vi "OnDataChange.vi"(0 "DemoStepMotor in":refnum<class "DemoStepMotor.lvclass">, 1 "DataExchange":T1, 3 "error in (no error)":errorcluster) -> (7 "DemoStepMotor out":refnum<class "DemoStepMotor.lvclass">, 10 "error out":errorcluster)   [LabVIEW 2020, in "DemoStepMotor.lvlib" / "DemoStepMotor.lvclass"]
uses:
  DemoStepMotor.lvclass
  Hardware Abstraction Layer/Component/Device/Device/DataExchange.ctl
  <vilib>/vision/Image Controls.llb/IMAQ Image.ctl
  DemoStepMotor.lvclass/DemoStepMotor.ctl
  Interface/DataListener Messages/OnDataChange Msg/OnDataChange Msg.lvclass/OnDataChange Msg.ctl
  <vilib>/ActorFramework/Message Enqueuer/Message Enqueuer.lvclass/Message Enqueuer.ctl
  <vilib>/ActorFramework/Message Enqueuer/Enqueue.vi
  Interface/DataListener Messages/OnDataChange Msg/OnDataChange Msg.lvclass
  C:/Program Files/National Instruments/LabVIEW 2020/vi.lib/ActorFramework/Message/Message.lvclass
  <vilib>/ActorFramework/Message Priority Queue/Priority Enqueue.vi
  Hardware Abstraction Layer/Component/Stage/Stage/Stage.lvclass
  Interface/DataListener/DataListener.lvclass
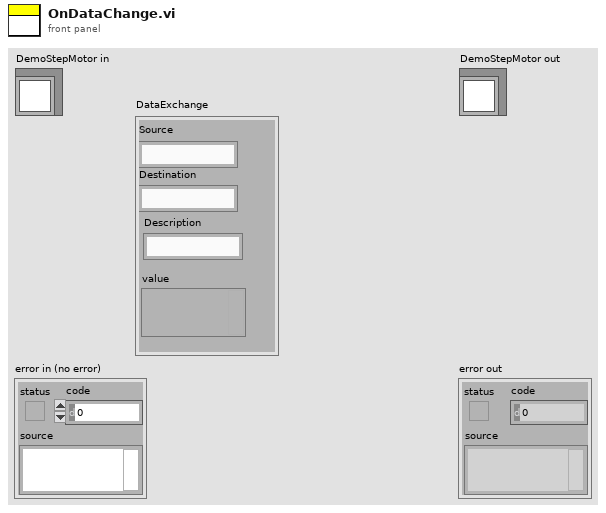
[diagram p1: front panel]
types:
  T1 = typedef "DataListener.lvclass/DataExchange.ctl" = cluster{"Source":string, "Destination":string, "Description":string, "value":variant}
  T2 = typedef "IMAQ Image.ctl" = refnum<image>
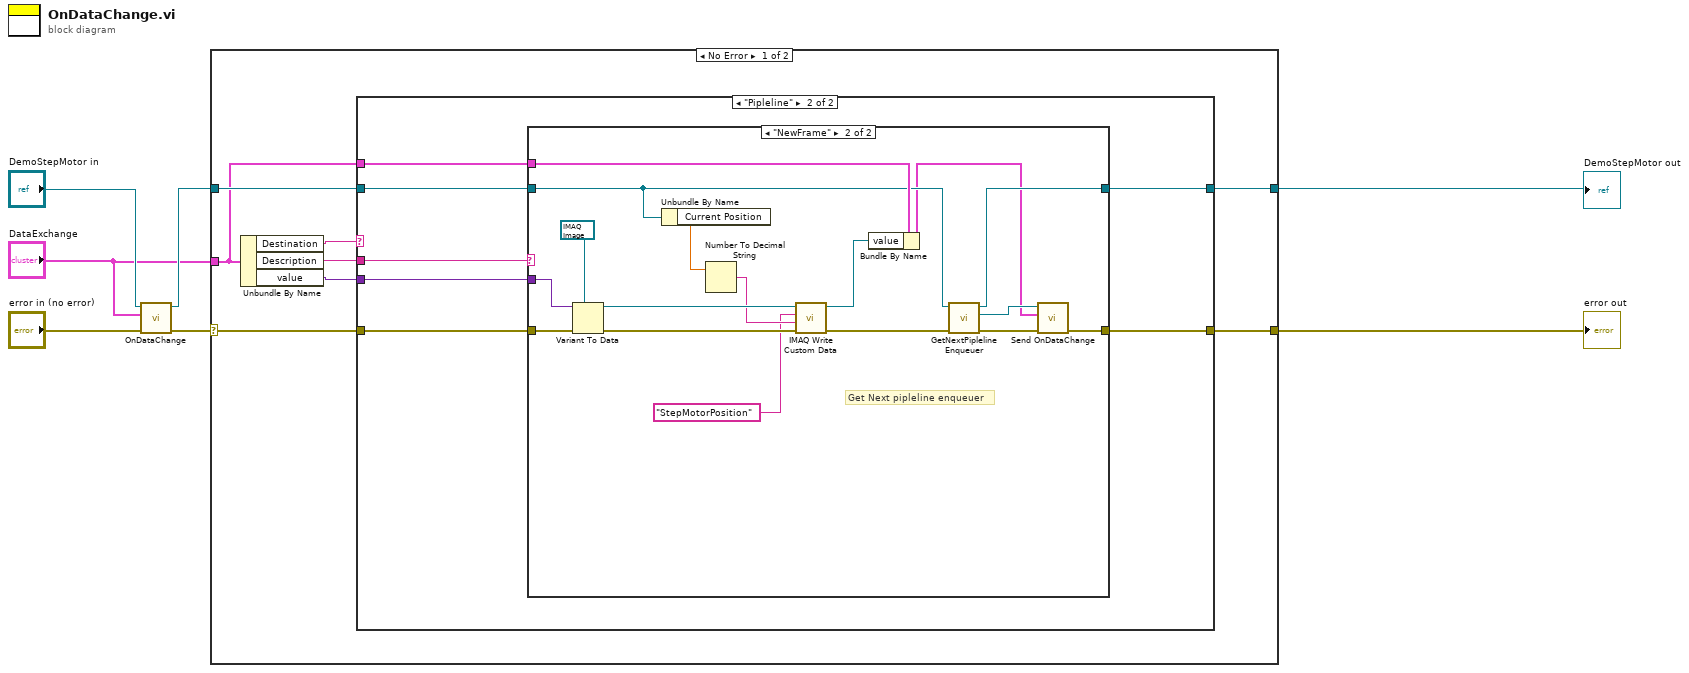
[diagram p0: block diagram]
diagram:
  n1 = call-parent "OnDataChange.vi"("Device in"="DemoStepMotor in", "DataExchange"="DataExchange", "error in (no error)"="error in (no error)") -> ("Device out"=w3:refnum<class "DemoStepMotor.lvclass">, "error out"=w5:errorcluster)  [unwired: 6 in]
  n2 = case shown="No Error" w5 {
    selector: w5 -> [w11 w45]
    tunnel: [w12 w45] -> w4
    tunnel: w3 -> [w14 w44]
    tunnel: [w13 w44] -> w2
    tunnel: "DataExchange" -> [w8 _]
    frame No Error {
      n3 = Unbundle By Name(w8) -> ("Destination"=w15:string, "Description"=w10:string, "value"=w9:variant)
      n4 = case shown="\"Pipleline\"" w15 {
        tunnel: [w17 w22] -> w13
        tunnel: w14 -> [w17 w21]
        tunnel: [w16 w19] -> w12
        tunnel: w11 -> [w16 w20]
        tunnel: w10 -> [_ w24]
        tunnel: w9 -> [_ w23]
        tunnel: w8 -> [_ w18]
        frame Default {
        }
        frame "Pipleline" {
          n5 = case shown="\"NewFrame\"" w24 {
            tunnel: w23 -> [_ w42]
            tunnel: [w26 w31] -> w22
            tunnel: w21 -> [w26 w32]
            tunnel: [w25 w28] -> w19
            tunnel: w20 -> [w25 w43]
            tunnel: w18 -> [_ w34]
            frame Default {
            }
            frame "NewFrame" {
              # "Get Next pipleline enqueuer"
              n6 = Variant To Data(error in=w43, type=T2 refnum ("New Image"), Variant=w42) -> (data=w40:T2, error out=w39:errorcluster)
              n7 = Unbundle By Name(w32) -> ("Current Position"=w37:dbl)
              n8 = Number To Decimal String(number=w37) -> (decimal integer string=w36:string)  [unwired: 1 in]
              n9 = call "IMAQ Write Custom Data"("error in (no error)"=w39, "Custom Data In"=w36, "Key"="StepMotorPosition", "Image"=w40) -> ("error out"=w38:errorcluster, "Image Out"=w33:T2)  [unwired: 6 in]
              n10 = Bundle By Name(cluster=w34, "value"=w33) -> (w27:T1)
              n11 = call-dynamic "GetNextPiplelineEnqueuer.vi"("error in (no error)"=w38, "Device in"=w32) -> ("error out"=w29:errorcluster, "NextPiplelineEnqueuer"=w30:refnum<class "Message Enqueuer.lvclass">, "Device out"=w31:refnum<class "DemoStepMotor.lvclass">)  [unwired: 7 in]
              n12 = call "Send OnDataChange.vi"("error in (no error)"=w29, "DataExchange"=w27, "Message Enqueuer"=w30) -> ("error out"=w28:errorcluster)  [unwired: 7 in, 1 out]
            }
          }
        }
      }
    }
    frame Error {
    }
  }
  "error out" <- w4
  "DemoStepMotor out" <- w2
